vi "Array.vi"() -> ()   [LabVIEW 2021]
panel:
  in  "Index":i32
  out "Element":dbl
  out "Size":dbl
  out "Slide":dbl[](array[slide]) scale=0.0..10.0
  in  "Array":dbl[](array[numeric])
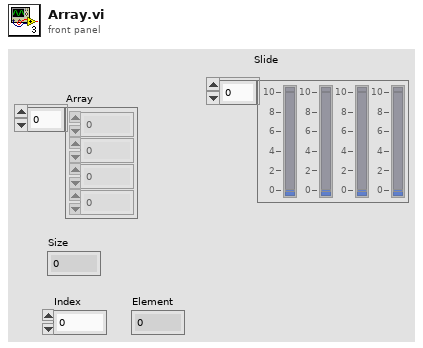
[diagram p1: front panel]
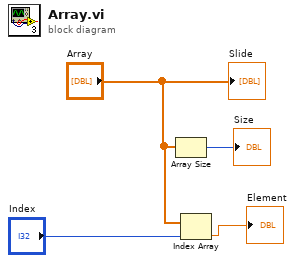
[diagram p0: block diagram]
diagram:
  n1 = Array Size(array="Array") -> (size(s)=→"Size":i32)
  n2 = Index Array(array="Array", index="Index") -> (element=→"Element":dbl)
  "Slide" <- "Array"
